vi "v1h_get_NC_var.vi"(3 "error in (no error)":errorcluster caption="错误输入（无错误）", 4 "NC_dimarray":cluster{"name":string, "size":u64}[](array[cluster]), 5 "refnum in":refnum<file>) -> (0 "error out":errorcluster caption="错误输出", 1 "NC_var":T1 {"NC_attrarray"."nc_type" items=["NC_NAT", "NC_BYTE", "NC_CHAR", "NC_SHORT", "NC_INT", "NC_FLOAT", "NC_DOUBLE"]}, 2 "refnum out":refnum<file>)   [LabVIEW 2016]
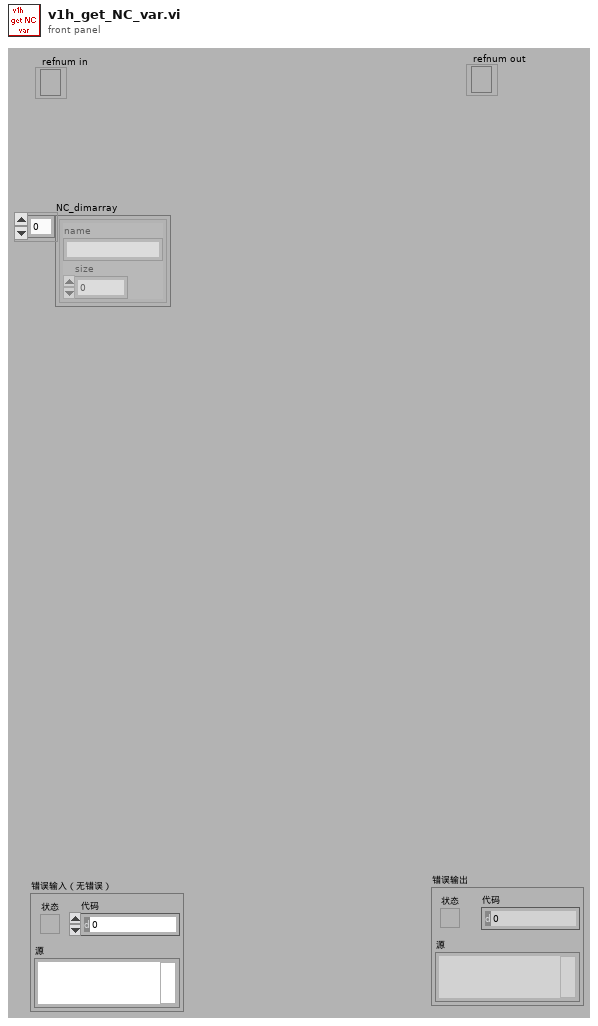
[diagram p1: front panel]
types:
  T1 = cluster{"xsz":u64, "shape":u64[], "dsizes":u64[], "name":string, "dimids":u64[], "NC_attrarray":cluster{"xsz":u64, "name":string, "nc_type":u16, "nelems":u64, "xvalue":string}[], "nc_type":enum16{"NC_NAT", "NC_BYTE", "NC_CHAR", "NC_SHORT", "NC_INT", "NC_FLOAT", "NC_DOUBLE"}, "len":u64, "begin":u64}
  T2 = cluster{"xsz":u64, "name":string, "nc_type":u16, "nelems":u64, "xvalue":string}[]
  T3 = cluster{"sz":u64, u64[], u64[], "NC_string":string, i32[], "NC_attrarray":cluster{"xsz":u64, "name":string, "nc_type":u16, "nelems":u64, "xvalue":string}[], "int32":i32, "int32":i32, "int32":i32}
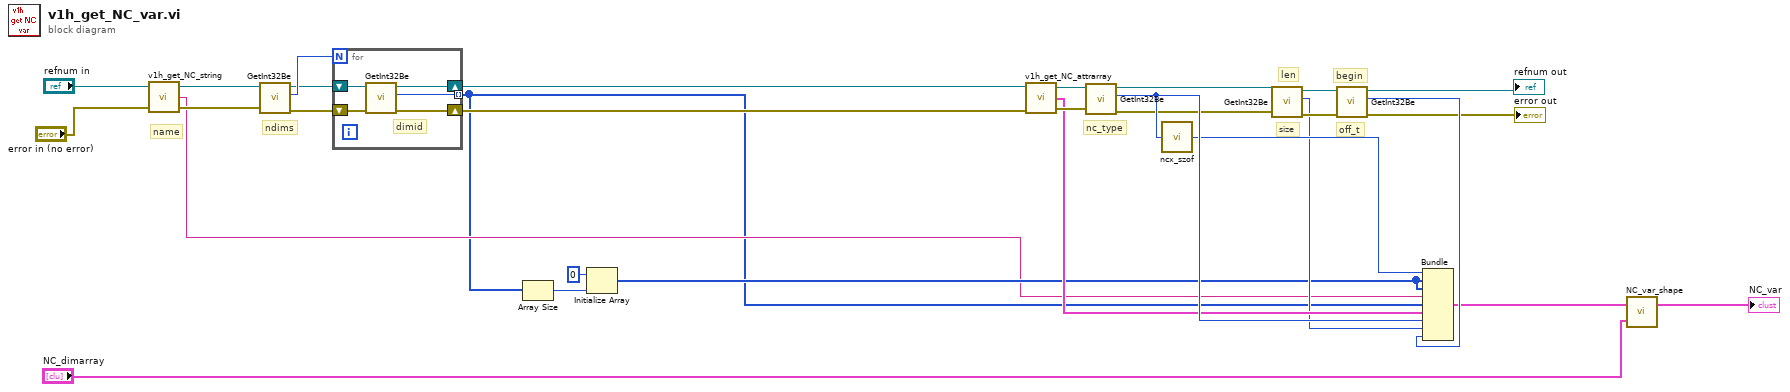
[diagram p0: block diagram]
diagram:
  # "begin"
  # "len"
  # "name"
  # "off_t"
  # "size"
  # "nc_type"
  # "ndims"
  n1 = call "v1h_get_NC_string.vi"("error in (no error)"="error in (no error)", "refnum in"="refnum in") -> ("error out"=w15:errorcluster, "NC_string"=w5:string, "refnum out"=w19:refnum<file>)  [unwired: 1 out]
  n2 = call "GetInt32Be.vi"("error in (no error)"=w15, "refnum in"=w19) -> ("error out"=w17:errorcluster, "int32"=w30:i32, "refnum out"=w20:refnum<file>)  [unwired: 3 out]
  n3 = for {
    N: w30 -> [_]
    shift-right: [w34] -> w25
    shift-left: w20 -> [w35]
    tunnel: [w33] -> w4 mode=indexing
    shift-right: [w31] -> w14
    shift-left: w17 -> [w32]
    # "dimid"
    n4 = call "GetInt32Be.vi"("error in (no error)"=w32, "refnum in"=w35) -> ("error out"=w31:errorcluster, "int32"=w33:i32, "refnum out"=w34:refnum<file>)  [unwired: 3 out]
  }
  n5 = Array Size(array=w4) -> (size(s)=w6:i32)
  n6 = Initialize Array(u64 0 ("size"), w6) -> (w7:u64[])
  n7 = call "v1h_get_NC_attrarray.vi"("error in (no error)"=w14, "refnum in"=w25) -> ("error out"=w11:errorcluster, "NC_attrarray"=w10:T2, "refnum out"=w26:refnum<file>)  [unwired: 1 in]
  n8 = call "GetInt32Be.vi"("error in (no error)"=w11, "refnum in"=w26) -> ("error out"=w12:errorcluster, "int32"=w28:i32, "refnum out"=w21:refnum<file>)  [unwired: 3 out]
  n9 = call "ncx_szof.vi"("nc_type"=w28) -> ("sz"=w27:u64)
  n10 = call "GetInt32Be.vi"("error in (no error)"=w12, "refnum in"=w21) -> ("error out"=w13:errorcluster, "int32"=w9:i32, "refnum out"=w22:refnum<file>)  [unwired: 3 out]
  n11 = call "GetInt32Be.vi"("error in (no error)"=w13, "refnum in"=w22) -> ("error out"=→"error out":errorcluster, "int32"=w29:i32, "refnum out"=→"refnum out":refnum<file>)  [unwired: 3 out]
  n12 = Bundle("sz"=w27, w7, w7, "NC_string"=w5, w4, "NC_attrarray"=w10, "int32"=w28, "int32"=w9, "int32"=w29) -> (w2:T3)  [unwired: 1 out]
  n13 = call "NC_var_shape.vi"("NC_dimarray"="NC_dimarray", "NC_var in"=w2) -> ("NC_var out"=→"NC_var":T1)  [unwired: 1 out]
